vi "metadata operations.vi"(5 "add time?":bool, 6 "sw":u32, 7 "add to stack writer":bool, 8 "error in (no error)":errorcluster, 9 "value":dbl, 10 "key":string, 11 "Operation":T2(ring)) -> (0 "error out":errorcluster, 1 "spreadsheet table":string, 2 "Value Array":dbl[](array[numeric]), 3 "lookup table out":T1(array[cluster]))   [LabVIEW 2013]
uses:
  Image-Stack-Compressor/StackWriterWrapper/LV code/StackWriterWrapper.lvlib
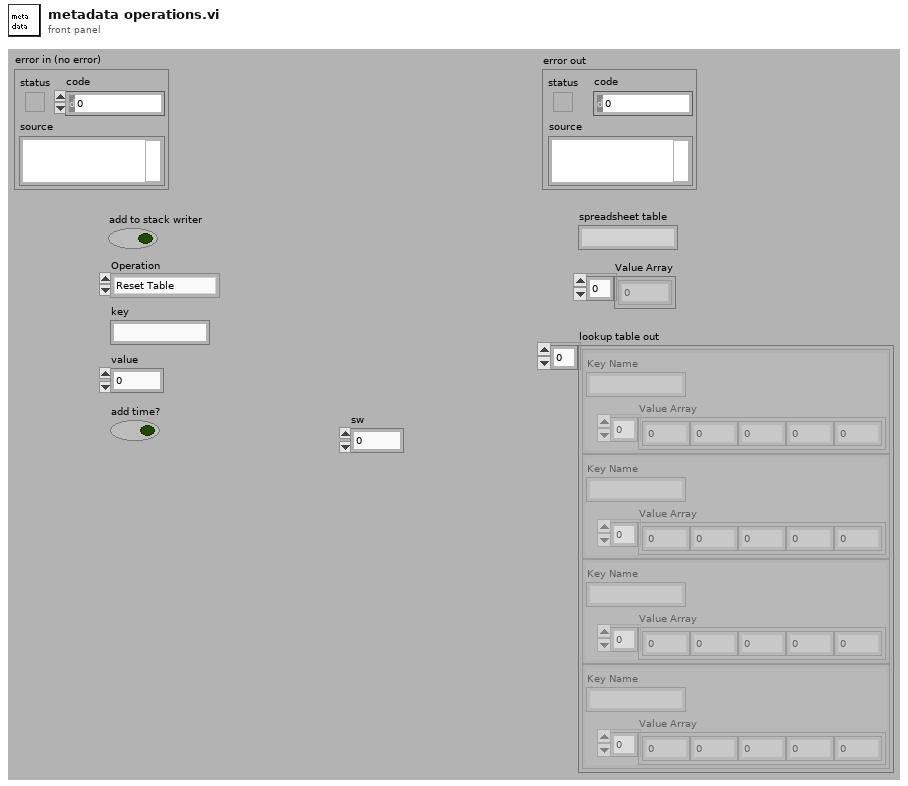
[diagram p1: front panel]
types:
  T1 = cluster{"Key Name":string, "Value Array":dbl[]}[]
  T2 = enum16{"Reset Table", "Get Values", "Add Value", "Get Table", "Get Spreadsheet", "set stack writer"}
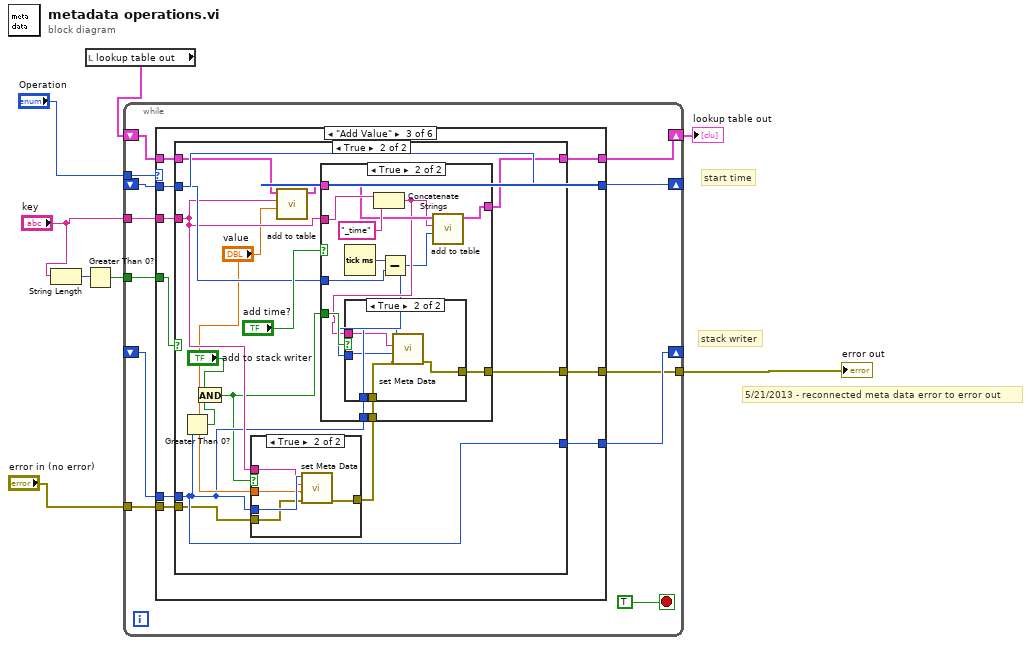
[diagram p0: block diagram]
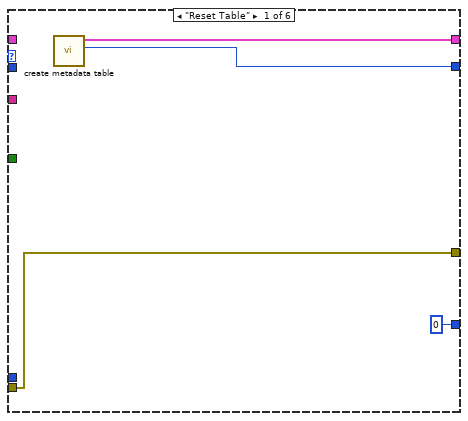
[diagram p2: hidden frame]
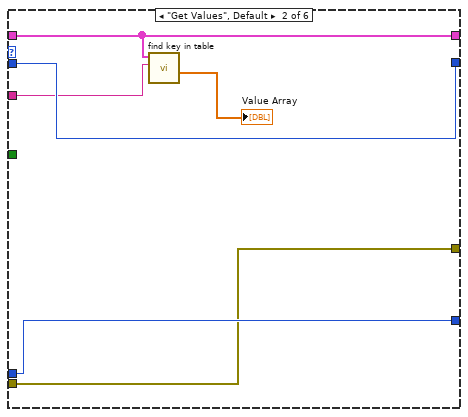
[diagram p3: hidden frame]
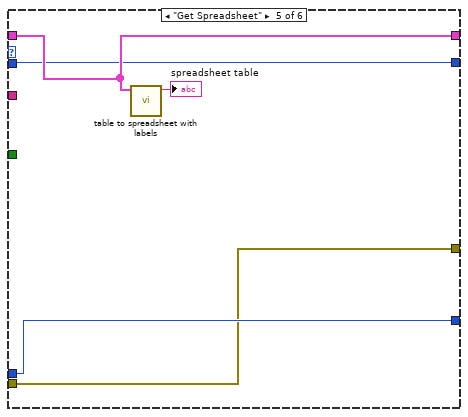
[diagram p9: hidden frame]
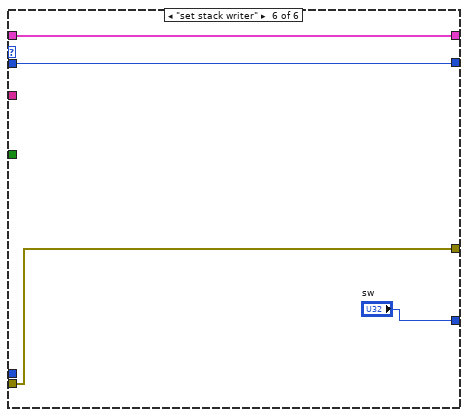
[diagram p10: hidden frame]
diagram:
  # "5/21/2013 - reconnected meta data error to error out"
  # "stack writer"
  # "start time"
  n1 = String Length(string="key") -> (length=w4:i32)
  n2 = Greater Than 0?(x=w4) -> (x > 0?=w3:bool)
  n3 = local read "lookup table out"() -> (w6:T1)
  n4 = while {
    shift-right: [w19] -> w7
    shift-left: w6 -> [w16]
    tunnel: "Operation" -> [w17]
    shift-right: [w18] -> _
    shift-left: _ -> [w15]
    tunnel: "key" -> [w14]
    tunnel: w3 -> [w13]
    shift-right: [w11] -> _
    shift-left: _ -> [w12]
    tunnel: [w10] -> w1
    tunnel: "error in (no error)" -> [w9]
    stop <- TRUE stop-if-true
    n5 = case shown="\"Add Value\"" w17 {
      tunnel: [w24 w28 w38 w86 w90 w93] -> w19
      tunnel: [w23 w30 w37 w85 w89 w94] -> w18
      tunnel: w16 -> [_ w28 w39 w86 w90 w93]
      tunnel: w15 -> [_ w30 w37 w85 w89 w94]
      tunnel: w14 -> [_ w29 w36 _ _ _]
      tunnel: w13 -> [_ _ w35 _ _ _]
      tunnel: w12 -> [_ w26 w34 w84 w88 _]
      tunnel: [u32 0 ("sw") w26 w33 w84 w88 "sw"] -> w11
      tunnel: [w21 w25 w32 w83 w87 w92] -> w10
      tunnel: w9 -> [w21 w25 w31 w83 w87 w92]
      frame "Reset Table" {
        n6 = call "create metadata table.vi"() -> ("start time"=w23:u32, "lookup table"=w24:T1)  [unwired: 10 in]
      }
      frame "Get Values", Default {
        n7 = call "find key in table.vi"("key"=w29, "lookup table"=w28) -> ("Value Array"=→"Value Array":dbl[])  [unwired: 7 in, 2 out]
      }
      frame "Add Value" {
        n8 = case shown="True" w35 {
          tunnel: w39 -> [w42 w56]
          tunnel: [w42 w53] -> w38
          tunnel: w37 -> [_ w52]
          tunnel: w36 -> [_ w51]
          tunnel: w34 -> [w41 w46]
          tunnel: [w41 w46] -> w33
          tunnel: [w40 w43] -> w32
          tunnel: w31 -> [w40 w44]
          frame False {
          }
          frame True {
            n9 = Greater Than 0?(x=w46) -> (x > 0?=w47:bool)
            n10 = And(x="add to stack writer", y=w47) -> (x .and. y?=w45:bool)
            n11 = case shown="True" w45 {
              tunnel: w51 -> [_ w61]
              tunnel: "value" -> [_ w60]
              tunnel: [w57 w59] -> w48
              tunnel: w46 -> [_ w62]
              tunnel: w44 -> [w57 w58]
              frame False {
              }
              frame True {
                n12 = call "set Meta Data.vi"("error in (no error)"=w58, "fieldvalue"=w60, "fieldname"=w61, "sw"=w62) -> ("error out"=w59:errorcluster)  [unwired: 5 in, 2 out]
              }
            }
            n13 = call "add to table.vi"("value"="value", "key"=w51, "lookup table"=w56) -> ("lookup table out"=w54:T1)  [unwired: 8 in]
            n14 = case shown="True" "add time?" {
              tunnel: w51 -> [_ w76]
              tunnel: w52 -> [_ w73]
              tunnel: w54 -> [w64 w72]
              tunnel: [w64 w71] -> w53
              tunnel: w45 -> [_ w70]
              tunnel: w48 -> [w63 w67]
              tunnel: w46 -> [_ w66]
              tunnel: [w63 w65] -> w43
              frame False {
              }
              frame True {
                n15 = Tick Count (ms)() -> (millisecond timer value=w74:u32)
                n16 = Concatenate Strings(w76, "_time" ("string")) -> (w69:string)
                n17 = Subtract(x=w74, y=w73) -> (x-y=w68:u32)
                n18 = case shown="True" w70 {
                  tunnel: w69 -> [_ w80]
                  tunnel: w68 -> [_ w79]
                  tunnel: w67 -> [w77 w82]
                  tunnel: w66 -> [_ w81]
                  tunnel: [w77 w78] -> w65
                  frame False {
                  }
                  frame True {
                    n19 = call "set Meta Data.vi"("error in (no error)"=w82, "fieldvalue"=w79, "fieldname"=w80, "sw"=w81) -> ("error out"=w78:errorcluster)  [unwired: 5 in, 2 out]
                  }
                }
                n20 = call "add to table.vi"("value"=w68, "key"=w69, "lookup table"=w72) -> ("lookup table out"=w71:T1)  [unwired: 8 in]
              }
            }
          }
        }
      }
      frame "Get Table" {
      }
      frame "Get Spreadsheet" {
        n21 = call "table to spreadsheet with labels.vi"("lookup table"=w90) -> ("spreadsheet table"=→"spreadsheet table":string)  [unwired: 10 in]
      }
      frame "set stack writer" {
      }
    }
  }
  "lookup table out" <- w7
  "error out" <- w1
